vi "Initialize.vi"(8 "error in (no error)":errorcluster, 11 "State in":T1={"State"=enum."Idle", "Start Time"=timestamp(0 s since 1904-01-01), "Current Time"=timestamp(0 s since 1904-01-01), "First Iteration"=FALSE, "Process Name"="", "Output Error"=FALSE, "Log Started"=FALSE, "Cycle Period"=50.0, "Configuration"={"Valve Settings"={"D-O Settings"={"DAQmx Task Name"="", "Output Channel"=0, "Output Channel Names"=[]}, "VICI Electronic Actuator"={"VISA resource name"="", "Mode"=enum."Two Positions With Stops", "Simulated"=FALSE}}, "Valve Type"=enum."Digital Output Valve", "Time On (Sec)"=0.0, "Time Off (Sec)"=0.0, "Run?"=FALSE}, "Data"={"D-O State"=enum."Off"}} {"Configuration"."Valve Settings"."D-O Settings"."Output Channel" items=["Choose a Channel"]}) -> (0 "error out":errorcluster, 1 "Initialized":bool, 3 "State out":T1={"State"=enum."Idle", "Start Time"=timestamp(0 s since 1904-01-01), "Current Time"=timestamp(0 s since 1904-01-01), "First Iteration"=FALSE, "Process Name"="", "Output Error"=FALSE, "Log Started"=FALSE, "Cycle Period"=50.0, "Configuration"={"Valve Settings"={"D-O Settings"={"DAQmx Task Name"="", "Output Channel"=0, "Output Channel Names"=[]}, "VICI Electronic Actuator"={"VISA resource name"="", "Mode"=enum."Two Positions With Stops", "Simulated"=FALSE}}, "Valve Type"=enum."Digital Output Valve", "Time On (Sec)"=0.0, "Time Off (Sec)"=0.0, "Run?"=FALSE}, "Data"={"D-O State"=enum."Off"}} {"Configuration"."Valve Settings"."D-O Settings"."Output Channel" items=["Choose a Channel"]})   [LabVIEW 2018, in "D-O Module.lvlib" / "D-O Module Engine.lvlib"]
uses:
  D-O Module Engine.lvlib
  State Cluster.ctl
  State Enum.ctl
  Valve Clusters.ctl
  D-O Module Settings Cluster.ctl
  D-O Device Settings Cluster.ctl
  VICI Electronic Actuator/VICI Electronic Actuator Settings.ctl
  Tag VIs/Tag FGV Operation Enum.ctl
  Shared Variables/Dynamic Shared Variables.lvlib
  DIO Valve/VICI Electronic Actuator.lvlib
  D-O Module.lvlib
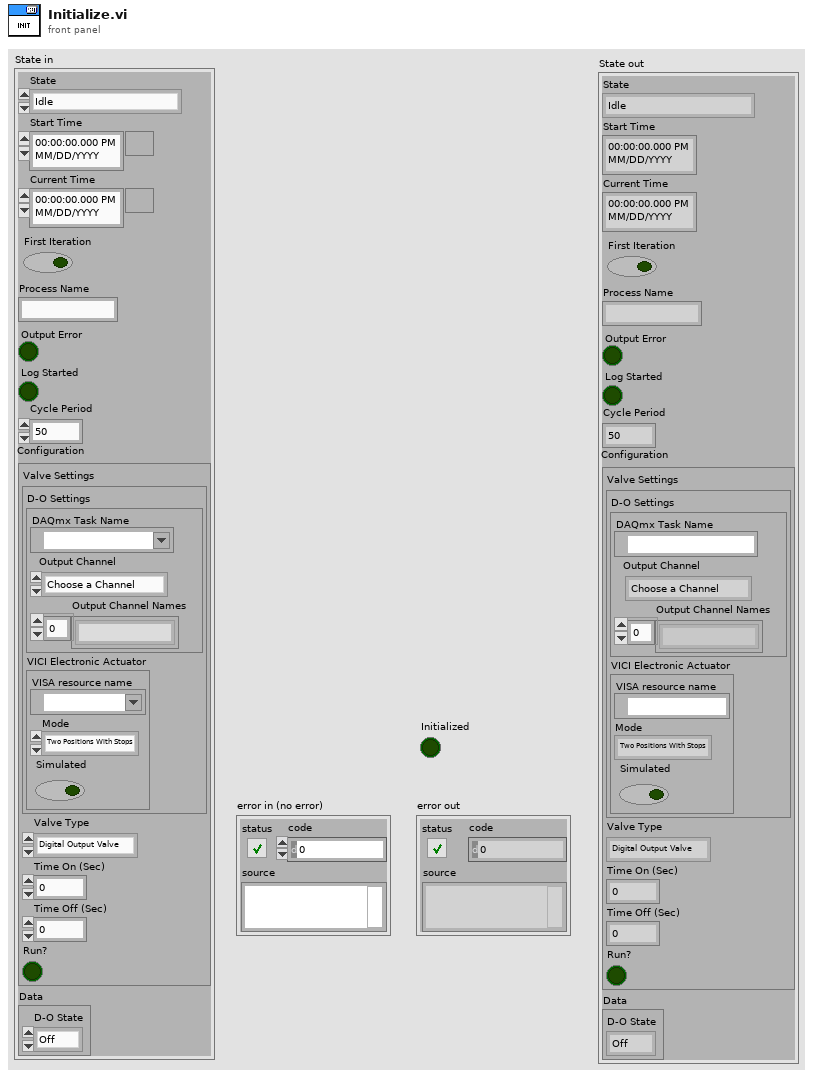
[diagram p1: front panel]
types:
  T1 = typedef "D-O Module.lvlib/D-O Module Engine.lvlib/State Cluster.ctl" = cluster{"State":T2, "Start Time":timestamp, "Current Time":timestamp, "First Iteration":bool, "Process Name":string, "Output Error":bool, "Log Started":bool, "Cycle Period":dbl, "Configuration":T3, "Data":cluster{"D-O State":enum16{"Off", "On", "Not Initialized"}}}
  T2 = typedef "D-O Module.lvlib/D-O Module Engine.lvlib/State Enum.ctl" = enum16{"Measuring", "Idle", "Paused"}
  T3 = typedef "D-O Module.lvlib/Valve Clusters.ctl" = cluster{"Valve Settings":T4, "Valve Type":enum16{"Default", "Digital Output Valve", "VICI Electronic Actuator"}, "Time On (Sec)":dbl, "Time Off (Sec)":dbl, "Run?":bool}
  T4 = typedef "D-O Module.lvlib/D-O Module Settings Cluster.ctl" = cluster{"D-O Settings":T5, "VICI Electronic Actuator":T6}
  T5 = typedef "D-O Module.lvlib/D-O Device Settings Cluster.ctl" = cluster{"DAQmx Task Name":refnum<k21>, "Output Channel":u16, "Output Channel Names":string[]}
  T6 = typedef "VICI Electronic Actuator.lvlib/VICI Electronic Actuator Settings.ctl" = cluster{"VISA resource name":refnum<visa-resource-name>, "Mode":enum16{"Two Positions With Stops", "Two Positions Without Stops", "Mutiposition"}, "Simulated":bool}
  T7 = typedef "Tag FGV Operation Enum.ctl" = enum16{"Init", "Set Notification Queue", "Create Tag", "Commit", "Write Tag (Numeric)", "Write Tag (Boolean)", "Read All Tags", "Read One Tag", "Delete Tag Category", "Set Alarm Parameters (Numeric)", "Set Alarm Parameters (Boolean)", "Enable All Alarms", "Disable All Alarms", "Delete All Tags", "Read Alarms", "Ack Alarm", "Read Alarm Parameters (Numeric)", "Read Alarm Parameters (Boolean)"}
  T8 = enum16{"Default", "Digital Output Valve", "VICI Electronic Actuator"}
  T9 = typedef "D-O Module.lvlib/D-O Module Tag Names Cluster.ctl" = cluster{"D-O Status":string, "Identifier Tag":string}
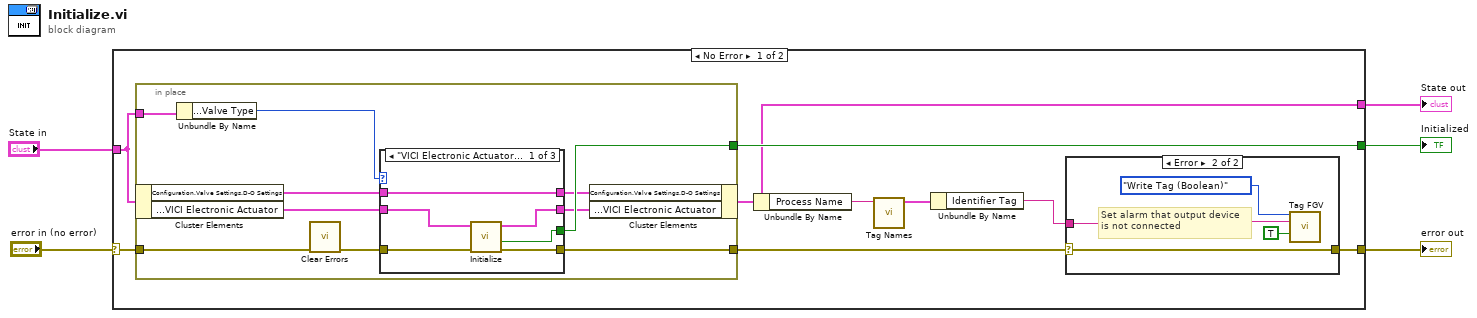
[diagram p0: block diagram]
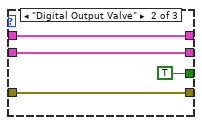
[diagram p2: hidden frame]
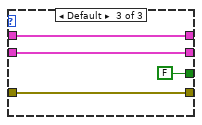
[diagram p3: hidden frame]
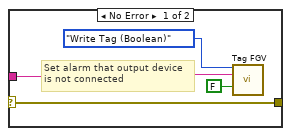
[diagram p4: hidden frame]
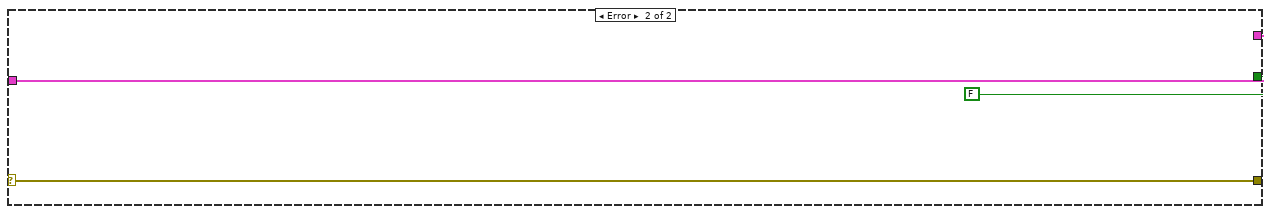
[diagram p5: hidden frame]
diagram:
  n1 = case shown="No Error" "error in (no error)" {
    selector: "error in (no error)" -> [w9 w49]
    tunnel: [w8 w49] -> w4
    tunnel: "State in" -> [w7 w48]
    tunnel: [w6 w48] -> w2
    tunnel: [w10 FALSE ("Initialized")] -> w1
    frame No Error {
      n2 = in-place {
        in-place-border: w7 -> [w24]
        in-place-border: [w22] -> w14
        in-place-border: [w20] -> w10
        in-place-border: w9 -> [w19]
        n3 = in-place-cluster #1(w7) -> ("Configuration.Valve Settings.D-O Settings"=w18:T5, "Configuration.Valve Settings.VICI Electronic Actuator"=w17:T6)
        n4 = Unbundle By Name(w24) -> ("Configuration.Valve Type"=w21:T8)
        n5 = call <vilib>:"Clear Errors.vi"("error in (no error)"=w19) -> ("error out"=w23:errorcluster)  [unwired: 5 in, 1 out]
        n6 = case shown="\"VICI Electronic Actuator\"" w21 {
          tunnel: w18 -> [w30 w34 w38]
          tunnel: [w30 w34 w38] -> w16
          tunnel: w23 -> [w26 w33 w37]
          tunnel: [w25 w33 w37] -> w22
          tunnel: [w27 TRUE ("Initialized") FALSE ("Initialized")] -> w20
          tunnel: w17 -> [w29 w31 w35]
          tunnel: [w28 w31 w35] -> w15
          frame "VICI Electronic Actuator" {
            n7 = call "Initialize.vi"("error in (no error)"=w26, "VICI Electronic Actuator In"=w29) -> ("error out"=w25:errorcluster, "Initialized"=w27:bool, "VICI Electronic Actuator Out"=w28:T6)  [unwired: 6 in, 1 out]
          }
          frame "Digital Output Valve" {
          }
          frame Default {
          }
        }
        n8 = in-place-cluster #1("Configuration.Valve Settings.D-O Settings"=w16, "Configuration.Valve Settings.VICI Electronic Actuator"=w15) -> (w6:T1)
      }
      n9 = Unbundle By Name(w6) -> ("Process Name"=w12:string)
      n10 = call "Tag Names.vi"("Process Name"=w12) -> ("Pump Module Tag Names"=w11:T9)  [unwired: 8 in, 2 out]
      n11 = Unbundle By Name(w11) -> ("Identifier Tag"=w13:string)
      n12 = case shown="Error" w14 {
        selector: w14 -> [w42 w46]
        tunnel: [w42 w46] -> w8
        tunnel: w13 -> [w39 w45]
        frame No Error {
          # "Set alarm that output device\nis not connected"
          n13 = call "Tag FGV.vi"("Operation"=Tag_FGV_Operation_Enum."Write Tag (Boolean)", "Tag Name"=w39, "Data"=FALSE) -> ()  [unwired: 5 in, 8 out]
        }
        frame Error {
          # "Set alarm that output device\nis not connected"
          n14 = call "Tag FGV.vi"("Operation"=Tag_FGV_Operation_Enum."Write Tag (Boolean)", "Tag Name"=w45, "Data"=TRUE) -> ()  [unwired: 5 in, 8 out]
        }
      }
    }
    frame Error {
    }
  }
  "error out" <- w4
  "State out" <- w2
  "Initialized" <- w1
